vi "report results.vi"(8 "error in":errorcluster, 10 "result":refnum<class "result.lvclass">, 11 "identifying queue reporter in":refnum<class "identifying queue reporter.lvclass">) -> (0 "error out":errorcluster, 3 "identifying queue reporter out":refnum<class "identifying queue reporter.lvclass">)   [LabVIEW 2015, in "identifying queue reporter.lvclass"]
uses:
  identifying queue reporter.lvclass
  result/result.lvclass
  result/result.lvclass/result.ctl
  message/communicator message.lvclass/communicator message.ctl
  identifying queue reporter.lvclass/identifying queue reporter.ctl
  communicator queue/identifying queue.lvclass/identifying queue.ctl
  result/get data ID.vi
  message/set sender.vi
  message/communicator message.lvclass
  communicator queue/identifying queue.lvclass
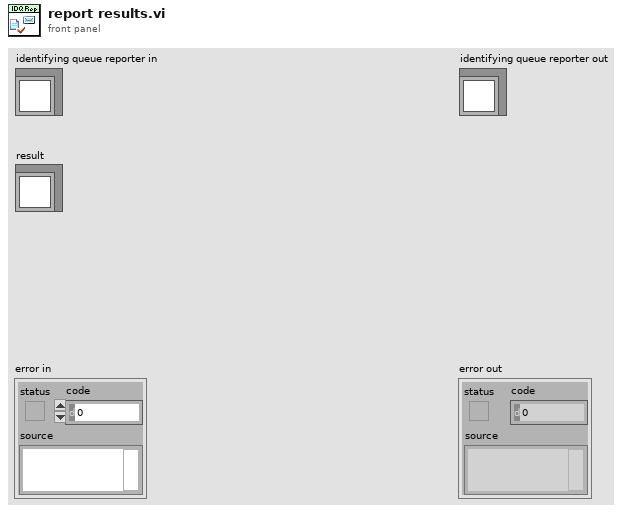
[diagram p1: front panel]
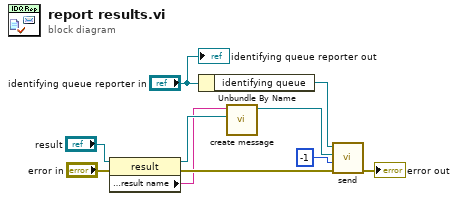
[diagram p0: block diagram]
diagram:
  n1 = property class="result"(reference="result", error in="error in") -> (reference out=w2:refnum<class "result.lvclass">, error out=w4:errorcluster, "accessors:result name"=w1:string)
  n2 = Unbundle By Name("identifying queue reporter in") -> ("identifying queue"=w9:refnum<class "identifying queue.lvclass">)
  n3 = call "create message.vi"("data"=w2, "ID"=w1) -> ("message"=w6:refnum<class "communicator message.lvclass">)  [unwired: 9 in]
  n4 = call "send.vi"("error in"=w4, "timeout in ms (-1)"=-1, "message"=w6, "message connection in"=w9) -> ("error out"=→"error out":errorcluster)  [unwired: 6 in, 1 out]
  "identifying queue reporter out" <- "identifying queue reporter in"
